vi "stateMachine_v2_Nov2015.vi"() -> ()   [LabVIEW 2014]
uses:
  daq_channel_read_parameter.ctl
  <vilib>/Platform/TimedLoop/XDataNode/timing_clust.ctl
  <vilib>/Platform/TimedLoop/XDataNode/nitl_modes.ctl
  <vilib>/Platform/TimedLoop/XDataNode/wakeup.ctl
  <vilib>/dex/Stream Element Allocation Mode.ctl
  states_def.ctl
  UDP_Para_def.ctl
  <vilib>/DAQmx/write.llb/DAQmx Write (Digital 1D Bool NChan 1Samp 1Line).vi
  <vilib>/platform/TimedLoop/XDataNode/XDataNode.xnode
  <vilib>/Platform/TimedLoop/XDataNode/XDNodeRunTimeDep.lvlib
  <resource>/objmgr/ni.dex.rc
panel:
  out "skipRewFlag":bool
  out "rightcounter":i32
  out "leftcounter":i32
  out "beh type":string
  out "vs type":string
  out "Tab Control":enum32{"State Machine"}(tab)
  in  "vsFilterPeriod_uS":i32=500 format="%#1.6f"
  in  "lickThreshold_V":fxp<+/-,16,5> format="%#.4g"
  in  "vsThreshold_V":fxp<+/-,16,5> format="%#.4g"
  in  "audioThreshold_V":fxp<+/-,16,5> format="%#.4g"
  in  "audioFilterPeriod_uS":i32=50000 format="%#1.6f"
  in  "audioOffState_V":fxp<+/-,16,5> format="%#.4g"
  out "rtFIFOsize":u32=50
  out "rtFIFOtimeout":u32
  out "rtFIFOdataPool":u32=50
  out "stateMachineCycle_uS":i64=500
  out "(Actual)":i64
  in  "delay_uS":u32
  out "IP_RT":string="192.168.137.2"
  in  "port_broadcast":u16=9091
  out "IP_host":string="192.168.137.1"
  out "port_host":u16=9090
  in  "Tab Control 2":enum32{"Data Transfer"}(tab)
  out "stream counter":u32
  out "Is Connected":bool
  out "Available Elements for Writing":i32
  out "stream writer buffer size":i32=500
  in  "rewardPeriod_uS":u32
  in  "waterOn_uS":u32
  in  "timeout_uS":u32=5000000
  in  "shockOn_uS":u32
  in  "Stop state":bool
  out "Initial data received":bool
  out "Tab Control 3":enum32{"Current status"}(tab)
  in  "toneReward":bool
  out "ABORT":bool
  out "trialStart":bool
  out "trialDone":bool
  out "Busy":bool
  out "stateLatched":bool
  out "curKey":u32=1
  out "curState":u32
  out "rtFIFOdataDim":i32
  in  "manualShock":bool
  in  "manualWaterRight":bool
  in  "manualWaterLeft":bool
  in  "lickReward":bool
  in  "allowPunish":bool
  in  "forceLRswitch":bool
  in  "allowCorrection":bool
  in  "allowAutoWater":bool
  out "error out":errorcluster
  in  "trialKey":i32[](array[numeric])
  in  "rwdrefPeriod_uS":u32
  out "FlagWaterLeft":bool
  in  "chanellParaCluster":T1={"audioOffState_V"=0.0, "audioFilterPeriod_uS"=50000, "audioThreshold_V"=0.0, "vsThreshold_V"=0.0, "vsFilterPeriod_uS"=0, "lickThreshold_V"=0.0} {"vsFilterPeriod_uS" format="%#1.6f"; "audioFilterPeriod_uS" format="%#1.6f"}
  out "leftWaterOnFlag":bool
  out "rightWaterOnFlag":bool
  out "contNoReward":i32
  out "rewardStatus":bool
types:
  T1 = typedef "daq_channel_read_parameter.ctl" = cluster{"audioOffState_V":fxp<+/-,16,5>, "audioFilterPeriod_uS":i32, "audioThreshold_V":fxp<+/-,16,5>, "vsThreshold_V":fxp<+/-,16,5>, "vsFilterPeriod_uS":i32, "lickThreshold_V":fxp<+/-,16,5>}
  T2 = typedef "XDNodeRunTimeDep.lvlib/timing_clust.ctl" = cluster{"Expected End [f-1]":u64, "Actual End [f-1]":u64, "Finished Late? [f-1]":bool, "Expected End [i-1]":u64, "Actual End [i-1]":u64, "Finished Late? [i-1]":bool, "Expected Start [i]":u64, "Actual Start [i]":u64, "Expected Start [f]":u64, "Actual Start [f]":u64, "Source Name":string, "Structure Name":string, "Period":i64, "Deadline":i64, "Offset":i64, "Start":i64, "Priority":i32, "Timeout":i32, "Mode":T3, "Wakeup Reason":T4, "Error":errorcluster, "Source Type":string, "Secondary Source Type":string, "Global End Time":u64, "Global Start Time":u64, "Frame Duration":u64, "Iteration Duration":u64, "Assigned CPU":i32, "I/O Scan Engine Mode":u32}
  T3 = typedef "XDNodeRunTimeDep.lvlib/nitl_modes.ctl" = enum32{"No Change", "Process missed periods, maintain original phase", "Discard missed periods, maintain original phase", "Process missed periods, ignore original phase", "Discard missed periods, ignore original phase"}
  T4 = typedef "XDNodeRunTimeDep.lvlib/wakeup.ctl" = enum32{"Normal", "Aborted", "Asynchronous wakeup", "Timing source error", "Timed loop error", "Timeout"}
  T5 = typedef "states_def.ctl" = enum16{"idle", "vs before", "vs", "vs after", "delay", "tone before", "tone", "tone after", "cycle end", "reward", "reward refractory", "punish", "punish refractory", "timeout", "exit", "manualwater"}
  T6 = typedef "Stream Element Allocation Mode.ctl" = u32
  T7 = typedef "UDP_Para_def.ctl" = enum16{"no", "start", "stop", "dly", "rwp", "rwf", "wdr", "shd", "tod", "lkr", "tlr", "alp", "msh", "mwl", "mwr", "alc", "lth", "vth", "ath", "aof", "afp", "vfp"}
  T8 = cluster{"leftLick":bool, "rightLick":bool, "visualStimuli2":bool, "tone":bool, "visualStimuli1":bool}
  T9 = cluster{"leftLick":dbl, "rightLick":dbl, "visualStimuli2":dbl, "tone":dbl, "visualStimuli1":dbl}
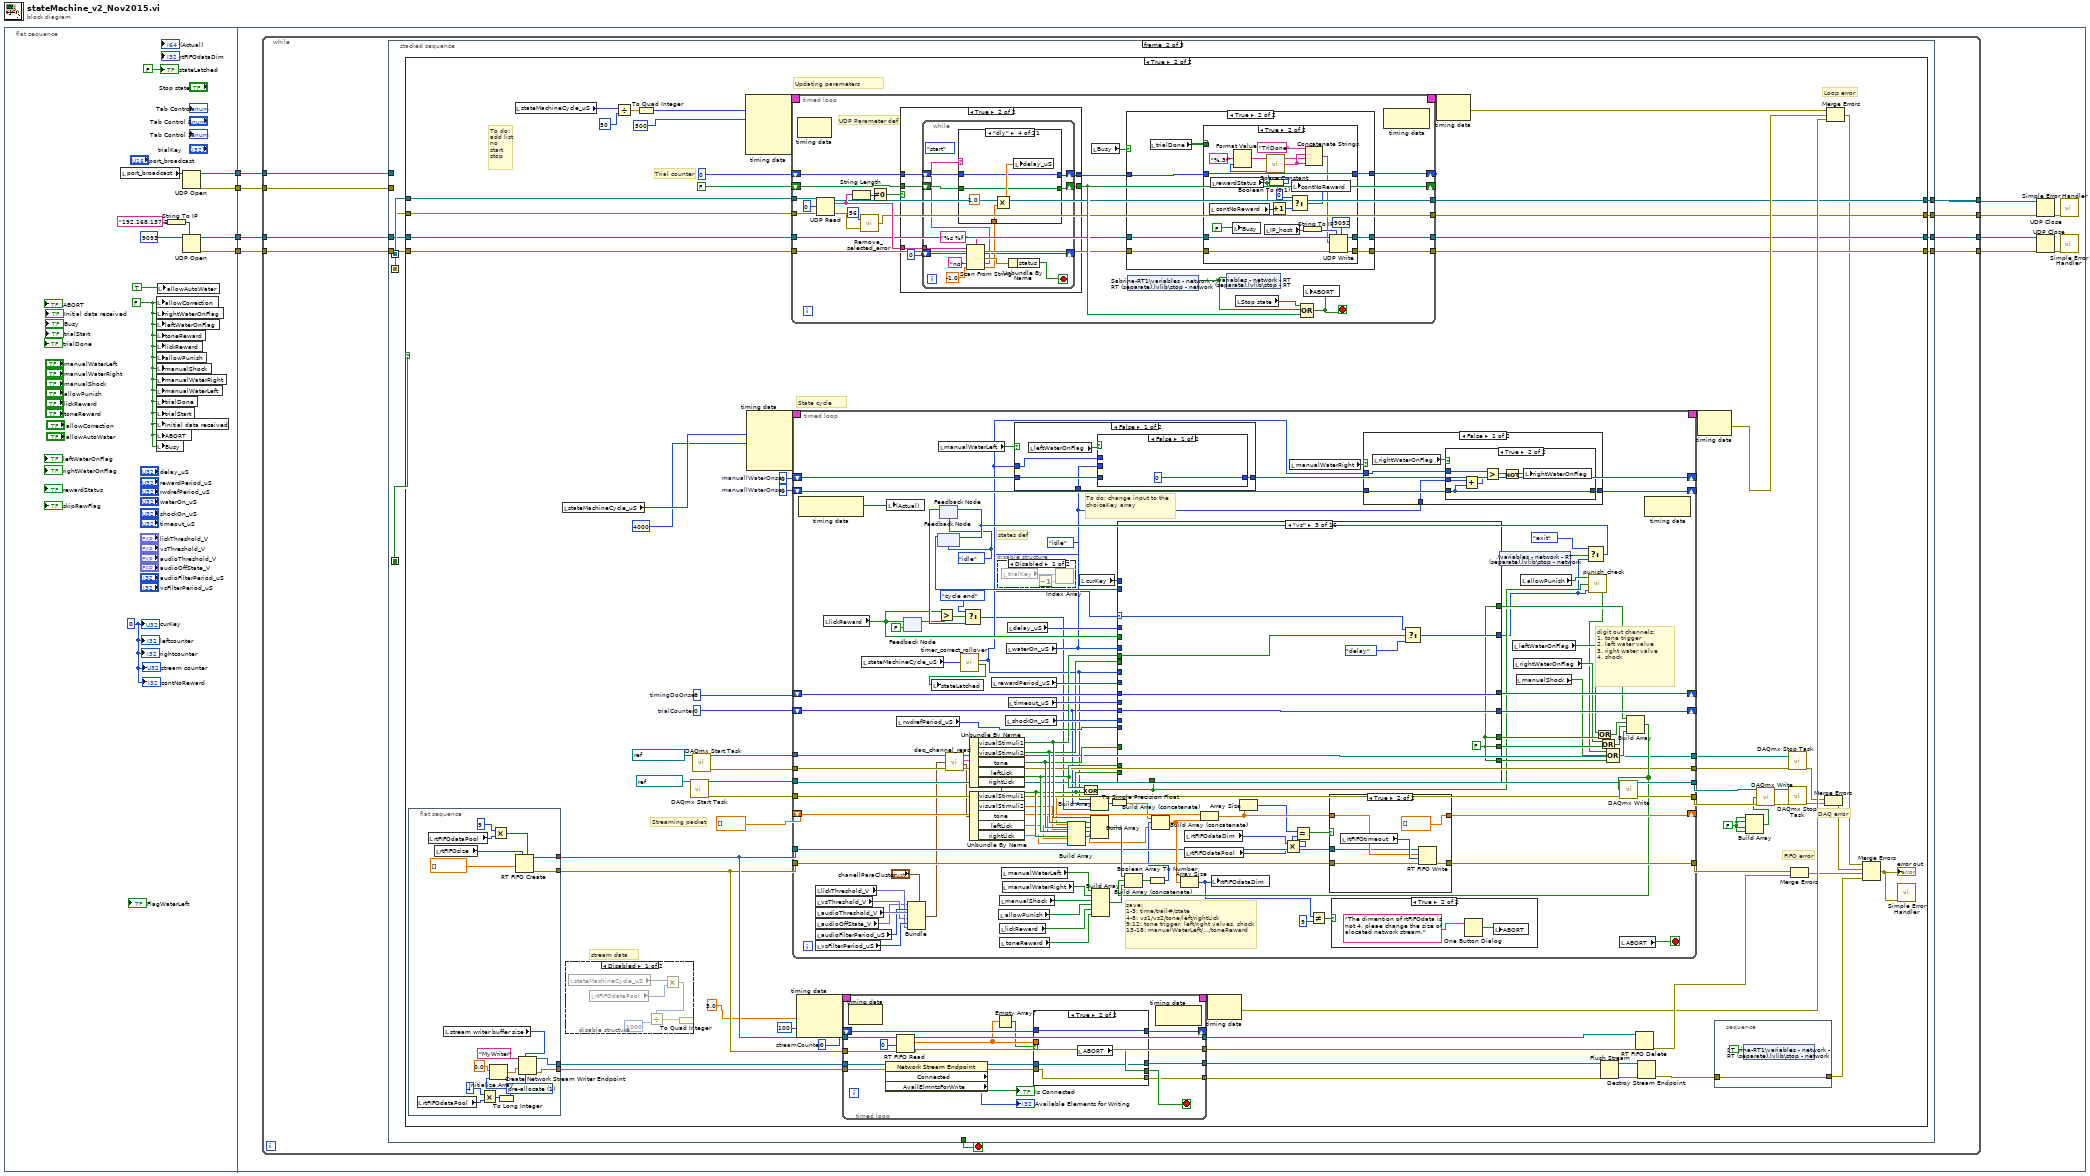
[diagram p0: block diagram]
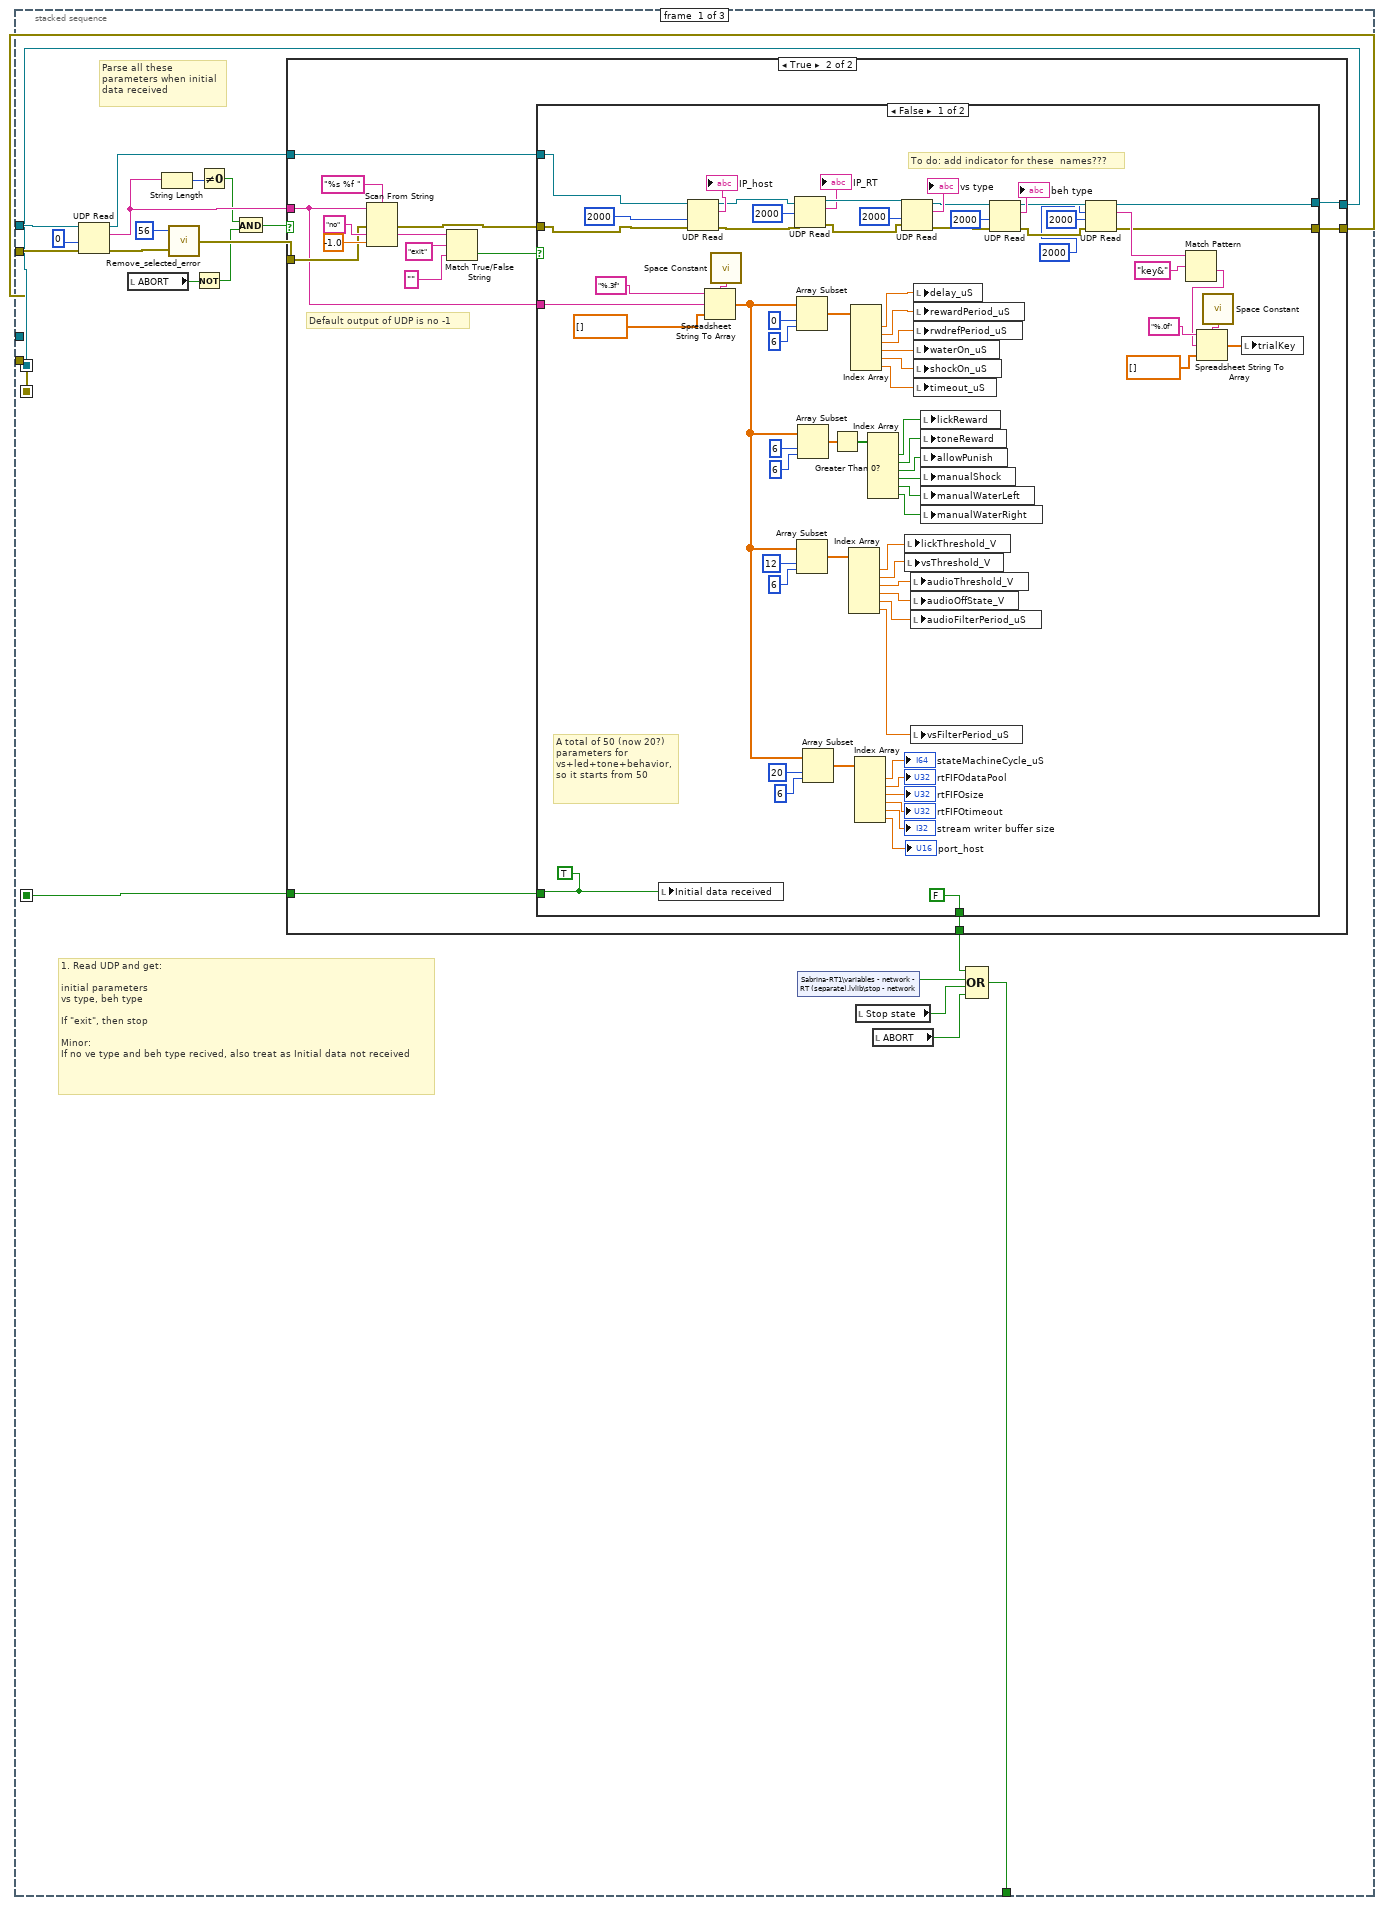
[diagram p2: hidden frame]
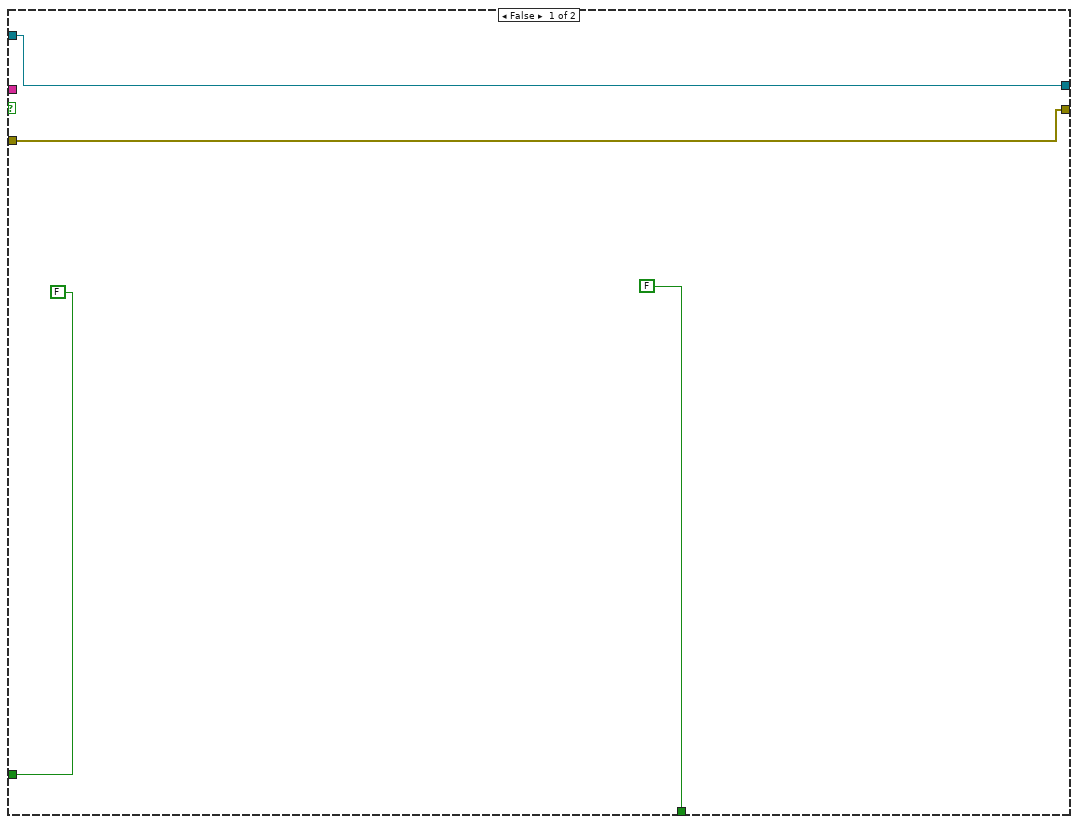
[diagram p3: hidden frame]
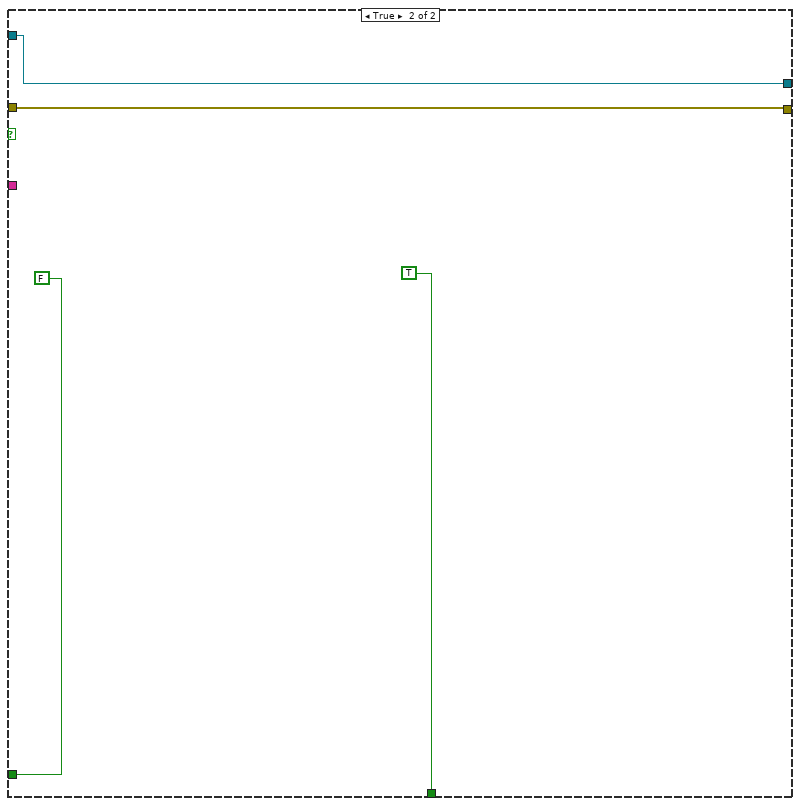
[diagram p4: hidden frame]
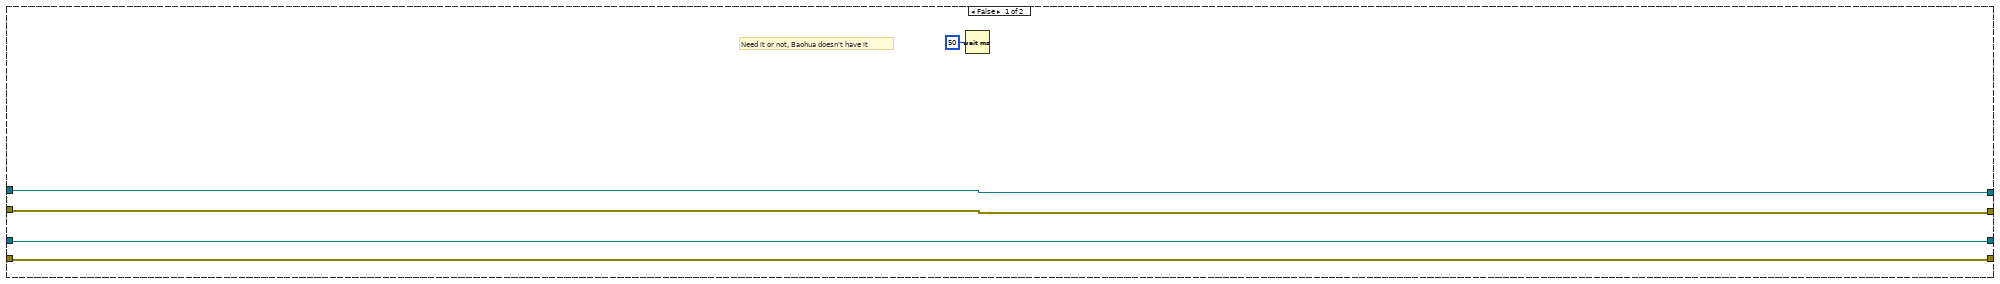
[diagram p5: hidden frame]
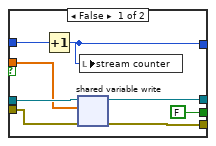
[diagram p7: hidden frame]
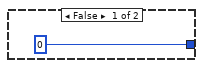
[diagram p9: hidden frame]
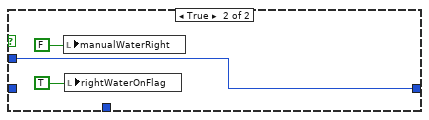
[diagram p10: hidden frame]
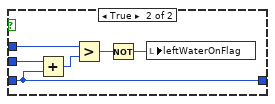
[diagram p11: hidden frame]
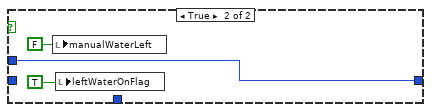
[diagram p12: hidden frame]
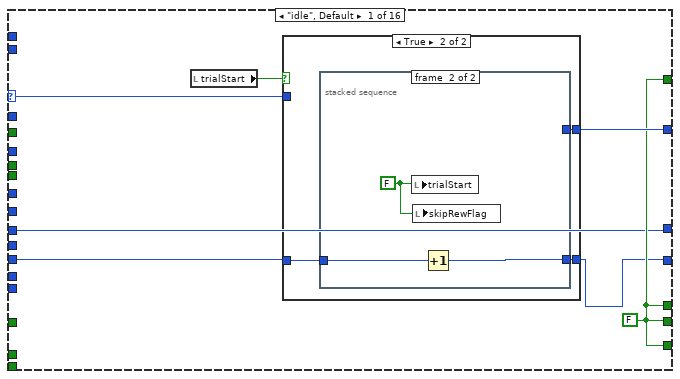
[diagram p15: hidden frame]
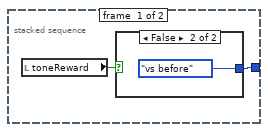
[diagram p17: hidden frame]
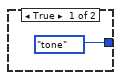
[diagram p18: hidden frame]
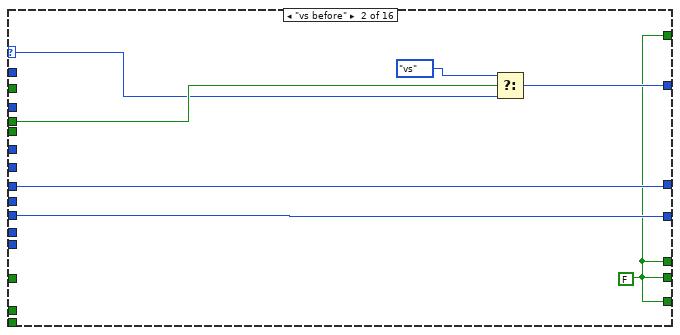
[diagram p19: hidden frame]
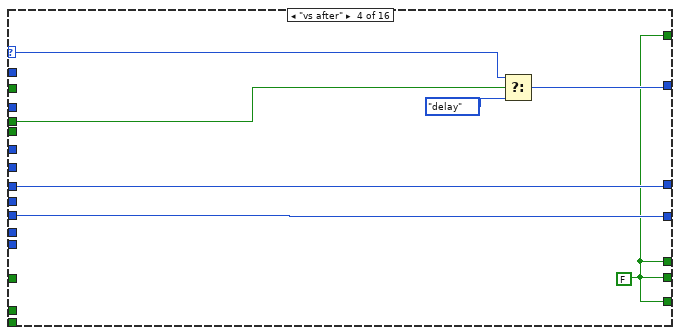
[diagram p20: hidden frame]
diagram:
  n1 = flat-sequence {
    tunnel: [w16] -> w4
    tunnel: [w15] -> w3
    tunnel: [w11] -> w2
    tunnel: [w10] -> w1
    tunnel: w4 -> [w26]
    tunnel: w3 -> [w25]
    tunnel: w2 -> [w21]
    tunnel: w1 -> [w20]
    frame #0 {
      w7 = FALSE
      w6 = 0
      n2 = local read "port_broadcast"() -> (w14:u16)
      n3 = local write "allowCorrection"(w7) -> ()
      n4 = local write "rightWaterOnFlag"(w7) -> ()
      n5 = local write "leftWaterOnFlag"(w7) -> ()
      n6 = local write "toneReward"(w7) -> ()
      n7 = local write "lickReward"(w7) -> ()
      n8 = local write "allowPunish"(w7) -> ()
      n9 = local write "manualShock"(w7) -> ()
      n10 = local write "manualWaterRight"(w7) -> ()
      n11 = local write "manualWaterLeft"(w7) -> ()
      n12 = local write "trialDone"(w7) -> ()
      n13 = local write "trialStart"(w7) -> ()
      n14 = local write "Initial data received"(w7) -> ()
      n15 = local write "ABORT"(w7) -> ()
      n16 = local write "Busy"(w7) -> ()
      n17 = local write "allowAutoWater"(TRUE) -> ()
      n18 = String To IP(1:"192.168.137.2") -> (0:w8:u32)
      n19 = UDP Open(7:w8, 11:u16 9093) -> (port=w11:refnum<k16>, 0:w10:errorcluster)  [unwired: 3 in, 1 out]
      n20 = UDP Open(11:w14) -> (port=w16:refnum<k16>, 0:w15:errorcluster)  [unwired: 4 in, 1 out]
      "stateLatched" <- FALSE
      "curKey" <- w6
      "leftcounter" <- w6
      "rightcounter" <- w6
      "stream counter" <- w6
      "contNoReward" <- w6
    }
    frame #1 {
      n21 = while {
        tunnel: w26 -> [w35]
        tunnel: w25 -> [w34]
        tunnel: [w32] -> w23
        tunnel: [w31] -> w22
        tunnel: w21 -> [w30]
        tunnel: w20 -> [w29]
        tunnel: [w28] -> w19
        tunnel: [w27] -> w18
        stop <- w33 stop-if-true
        n22 = stacked-sequence {
          seq-local: [w45 _ _] -> [_ w161 _]
          seq-local: [w37 _ _] -> [_ w158 _]
          seq-local: [w36 _ _] -> [_ w157 _]
          tunnel: w35 -> [w56 _ _]
          tunnel: w34 -> [w55 _ _]
          tunnel: [w46 _ _] -> w33
          tunnel: [_ w160 _] -> w32
          tunnel: [_ w159 _] -> w31
          tunnel: w30 -> [_ w156 _]
          tunnel: w29 -> [_ w153 _]
          tunnel: [_ w155 _] -> w28
          tunnel: [_ w154 _] -> w27
          frame #0 {
            # "Parse all these \nparameters when initial\ndata received"
            # "1. Read UDP and get:\n\ninitial parameters\nvs type, beh type\n\nIf \"exit\", then stop\n\nMinor:\nIf no ve type and beh type recived, also treat as Initial data not received"
            n23 = UDP Read(connection ID=w56, timeout ms (25000)=0, 8:w55) -> (data out=w53:string, error out=w43:errorcluster, 3:w54:refnum<k16>)  [unwired: 1 in, 2 out]
            n24 = local read "ABORT"() -> (w41:bool)
            n25 = String Length(string=w53) -> (length=w52:i32)
            n26 = call "Remove_selected_error.vi"("error in (no error)"=w43, "errorCode"=56 ("timeout ms (25000)")) -> ("error out"=w44:errorcluster)
            n27 = Not(x=w41) -> (.not. x?=w38:bool)
            n28 = Not Equal To 0?(x=w52) -> (x != 0?=w39:bool)
            n29 = And(x=w39, y=w38) -> (x .and. y?=w40:bool)
            n30 = case shown="True" w40 {
              tunnel: w53 -> [_ w65]
              tunnel: w54 -> [w58 w66]
              tunnel: w44 -> [w57 w73]
              tunnel: [FALSE w64] -> w50
              tunnel: [FALSE w63] -> w45
              tunnel: [w58 w62] -> w37
              tunnel: [w57 w61] -> w36
              frame False {
              }
              frame True {
                # "Default output of UDP is no -1"
                n31 = Scan From String(format string="%s %f ", input string=w65, error in=w73, default 1="no" ("default value 1"), default 2=sgl -1.0 ("default value 1")) -> (error out=w67:errorcluster, output 1=w72:string)  [unwired: 2 in, 2 out]
                n32 = Match True/False String(2:"" ("false string"), 3:"exit" ("true string"), 4:w72) -> (0:w68:bool)  [unwired: 1 out]
                n33 = case shown="False" w68 {
                  tunnel: w67 -> [w110 w150]
                  tunnel: w66 -> [w111 w149]
                  tunnel: w65 -> [w142 _]
                  tunnel: [FALSE TRUE] -> w64
                  tunnel: [w140 FALSE] -> w63
                  tunnel: [w77 w149] -> w62
                  tunnel: [w76 w150] -> w61
                  frame False {
                    w140 = TRUE
                    # "A total of 50 (now 20?) parameters for vs+led+tone+behavior, so it starts from 50"
                    # "To do: add indicator for these  names???"
                    n34 = local write "Initial data received"(w140) -> ()
                    n35 = UDP Read(connection ID=w111, timeout ms (25000)=2000, 8:w110) -> (data out=→"IP_host":string, error out=w109:errorcluster, 3:w107:refnum<k16>)  [unwired: 1 in, 2 out]
                    n36 = call <vilib>:"Space Constant.vi"() -> ("String"=w147:string)
                    n37 = Spreadsheet String To Array(delimiter (Tab)=w147, format string="%.3f", spreadsheet string=w142, array type (2D Dbl)=sgl[] []) -> (array=w118:sgl[])
                    n38 = UDP Read(connection ID=w107, timeout ms (25000)=2000, 8:w109) -> (data out=→"IP_RT":string, error out=w108:errorcluster, 3:w106:refnum<k16>)  [unwired: 1 in, 2 out]
                    n39 = Array Subset(array=w118, index=0 ("timeout ms (25000)"), length=6 ("timeout ms (25000)")) -> (w136:sgl[])
                    n40 = Array Subset(array=w118, index=12 ("timeout ms (25000)"), length=6 ("timeout ms (25000)")) -> (w132:sgl[])
                    n41 = Array Subset(array=w118, index=6 ("timeout ms (25000)"), length=6 ("timeout ms (25000)")) -> (w129:sgl[])
                    n42 = Array Subset(array=w118, index=20 ("timeout ms (25000)"), length=6 ("timeout ms (25000)")) -> (w119:sgl[])
                    n43 = Greater Than 0?(x=w129) -> (x > 0?=w128:bool[])
                    n44 = Index Array(array=w132) -> (element #1=w94:sgl, element #2=w93:sgl, element #3=w92:sgl, element #4=w91:sgl, element #5=w90:sgl, element #6=w89:sgl)  [unwired: 6 in]
                    n45 = Index Array(array=w136) -> (element #1=w100:sgl, element #2=w99:sgl, element #3=w98:sgl, element #4=w97:sgl, element #5=w96:sgl, element #6=w95:sgl)  [unwired: 6 in]
                    n46 = Index Array(array=w119) -> (element #1=→"stateMachineCycle_uS":sgl, element #2=→"rtFIFOdataPool":sgl, element #3=→"rtFIFOsize":sgl, element #4=→"rtFIFOtimeout":sgl, element #5=→"stream writer buffer size":sgl, element #6=→"port_host":sgl)  [unwired: 6 in]
                    n47 = Index Array(array=w128) -> (element #1=w127:bool, element #2=w126:bool, element #3=w125:bool, element #4=w124:bool, element #5=w123:bool, element #6=w122:bool)  [unwired: 6 in]
                    n48 = UDP Read(connection ID=w106, timeout ms (25000)=2000, 8:w108) -> (data out=→"vs type":string, error out=w139:errorcluster, 3:w138:refnum<k16>)  [unwired: 1 in, 2 out]
                    n49 = local write "lickThreshold_V"(w94) -> ()
                    n50 = local write "vsThreshold_V"(w93) -> ()
                    n51 = local write "audioThreshold_V"(w92) -> ()
                    n52 = local write "audioOffState_V"(w91) -> ()
                    n53 = local write "audioFilterPeriod_uS"(w90) -> ()
                    n54 = local write "vsFilterPeriod_uS"(w89) -> ()
                    n55 = local write "delay_uS"(w100) -> ()
                    n56 = local write "rewardPeriod_uS"(w99) -> ()
                    n57 = local write "rwdrefPeriod_uS"(w98) -> ()
                    n58 = local write "waterOn_uS"(w97) -> ()
                    n59 = local write "shockOn_uS"(w96) -> ()
                    n60 = local write "timeout_uS"(w95) -> ()
                    n61 = local write "lickReward"(w127) -> ()
                    n62 = local write "toneReward"(w126) -> ()
                    n63 = local write "allowPunish"(w125) -> ()
                    n64 = local write "manualShock"(w124) -> ()
                    n65 = local write "manualWaterLeft"(w123) -> ()
                    n66 = local write "manualWaterRight"(w122) -> ()
                    n67 = UDP Read(connection ID=w138, timeout ms (25000)=2000, 8:w139) -> (data out=→"beh type":string, error out=w86:errorcluster, 3:w87:refnum<k16>)  [unwired: 1 in, 2 out]
                    n68 = UDP Read(connection ID=w87, max size (548)=2000 ("timeout ms (25000)"), timeout ms (25000)=2000, 8:w86) -> (data out=w81:string, error out=w76:errorcluster, 3:w77:refnum<k16>)  [unwired: 2 out]
                    n69 = Match Pattern(string=w81, regular expression="key&") -> (after substring=w79:string)  [unwired: 1 in, 3 out]
                    n70 = call <vilib>:"Space Constant.vi"() -> ("String"=w84:string)
                    n71 = Spreadsheet String To Array(delimiter (Tab)=w84, format string="%.0f", spreadsheet string=w79, array type (2D Dbl)=dbl[] []) -> (array=w82:dbl[])
                    n72 = local write "trialKey"(w82) -> ()
                  }
                  frame True {
                  }
                }
              }
            }
            n73 = shared-variable "Sabrina-RT1\\variables - network - RT (separate).lvlib\\stop - network"() -> (w49:bool)  [unwired: 1 in, 1 out]
            n74 = local read "Stop state"() -> (w48:bool)
            n75 = local read "ABORT"() -> (w47:bool)
            n76 = Compound Arithmetic op=OR(w50, w49, w48, w47) -> (w46:bool)
          }
          frame #1 {
            n77 = case shown="True" w161 {
              tunnel: w158 -> [w165 w211]
              tunnel: w157 -> [w164 w210]
              tunnel: [w165 w183] -> w160
              tunnel: [w164 w184] -> w159
              tunnel: w156 -> [w163 w188]
              tunnel: w153 -> [w162 w187]
              tunnel: [w162 w186] -> w155
              tunnel: [w163 w185] -> w154
              frame False {
                # "Need it or not, Baohua doesn't have it"
                n78 = Wait (ms)(milliseconds to wait=u32 50) -> ()  [unwired: 1 out]
              }
              frame True {
                w167 = 0  # manuallWaterOnset
                w168 = 0  # manuallWaterOnset
                w194 = FALSE
                w223 = 0  # streamCounter
                w226 = 0  # timingDoOnset
                w225 = 0  # trialCounter
                # "Streaming packet"
                # "Trial counter"
                # "Loop error"
                # "DAQ error"
                # "FIFO error"
                # "Updating parameters"
                # "State cycle"
                # "To do:\nadd list\nno\nstart\nstop"
                # "stream data"
                n79 = flat-sequence {
                  tunnel: [w253] -> w228
                  tunnel: [w252] -> w227
                  tunnel: [w251] -> w214
                  tunnel: [w250] -> w213
                  frame #0 {
                    w257 = T6 1 items=["allocate as needed", "pre-allocate"] ("element allocation mode")
                    n80 = local read "rtFIFOdataPool"() -> (w248:u32)
                    n81 = local read "rtFIFOdataPool"() -> (w245:u32)
                    n82 = local read "rtFIFOsize"() -> (w259:u32)
                    n83 = local read "stream writer buffer size"() -> (w249:i32)
                    n84 = Multiply(x=u32 4, y=w248) -> (x*y=w243:u32)
                    n85 = Multiply(x=9, y=w245) -> (x*y=w244:u32)
                    n86 = To Long Integer(number=w243) -> (32bit integer=w242:i32)
                    n87 = Initialize Array(sgl 0.0, w242) -> (w256:sgl[])
                    n88 = RT FIFO Create(1:sgl[] [], 4:w259, 6:w244) -> (8:w251:refnum<k33>, 11:w250:errorcluster)  [unwired: 5 in, 1 out]
                    n89 = Create Network Stream Writer Endpoint(6:w257, 7:w249, 9:w256, 11:"MyWriter" ("writer name")) -> (0:w253:errorcluster, 3:w252:refnum<k21>)  [unwired: 3 in]
                  }
                }
                n90 = local read "stateMachineCycle_uS"() -> (w212:i64)
                n91 = local read "stateMachineCycle_uS"() -> (w222:i64)
                n92 = disable-structure shown="Disabled" {
                  frame Disabled {
                    n93 = local read "stateMachineCycle_uS"() -> (w237:i64)
                    n94 = local read "rtFIFOdataPool"() -> (w236:u32)
                    n95 = Multiply(x=w237, y=w236) -> (x*y=w238:i64)
                    n96 = Divide(x=w238, y=i64 1000) -> (x/y=w235:dbl)
                    n97 = To Quad Integer(1:w235) -> ()  [unwired: 1 out]
                  }
                  frame Enabled {
                  }
                }
                n98 = Divide(x=w212, y=i64 50) -> (x/y=w218:dbl)
                n99 = To Quad Integer(1:w218) -> (0:w217:i64)
                n100 = call <vilib>:"DAQmx Start Task.vi"("task/channels in"=refnum<k21> "digitWrite" ("digitWrite")) -> ("task out"=w180:refnum<k21>, "error out"=w179:errorcluster)  [unwired: 13 in]
                n101 = call <vilib>:"DAQmx Start Task.vi"("task/channels in"=refnum<k21> "analogRead" ("DAQmx Task Name")) -> ("task out"=w170:refnum<k21>, "error out"=w169:errorcluster)  [unwired: 13 in]
                n102 = node-c288(w217, 500 ("Priority")) -> (w234:T2)  [unwired: 3 in]
                n103 = node-c288(w222, 4000 ("Priority")) -> (w232:T2)  [unwired: 3 in]
                n104 = timed-loop {
                  timing: w234 -> [_]
                  timing-out: [_] -> w233
                  shift-right: [w743] -> _
                  shift-left: 0 ("timeout ms (25000)") -> [w745]
                  shift-right: [w739] -> _
                  shift-left: FALSE -> [w742]
                  tunnel: [w736] -> w185
                  tunnel: [w735] -> w186
                  tunnel: w211 -> [w734]
                  tunnel: w210 -> [w733]
                  tunnel: w188 -> [w727]
                  tunnel: w187 -> [w730]
                  tunnel: [w729] -> w184
                  tunnel: [w728] -> w183
                  stop <- w741 stop-if-true
                  # "UDP Parameter def"
                  n105 = node-c288() -> ()  [unwired: 1 in, 1 out]
                  n106 = UDP Read(connection ID=w734, timeout ms (25000)=0, 8:w733) -> (data out=w746:string, error out=w732:errorcluster, 3:w728:refnum<k16>)  [unwired: 1 in, 2 out]
                  n107 = String Length(string=w746) -> (length=w748:i32)
                  n108 = call "Remove_selected_error.vi"("error in (no error)"=w732, "errorCode"=56 ("timeout ms (25000)")) -> ("error out"=w729:errorcluster)
                  n109 = Not Equal To 0?(x=w748) -> (x != 0?=w747:bool)
                  n110 = case shown="True" w747 {
                    tunnel: w746 -> [_ w790]
                    tunnel: w745 -> [w784 w789]
                    tunnel: [w784 w788] -> w744
                    tunnel: w742 -> [w783 w787]
                    tunnel: [w783 w786] -> w739
                    frame False {
                    }
                    frame True {
                      n111 = while {
                        tunnel: w790 -> [w804]
                        shift-right: [w791] -> _
                        shift-left: 0 ("timeout ms (25000)") -> [w792]
                        shift-right: [w797] -> w788
                        shift-left: w789 -> [w798]
                        shift-right: [w795] -> w786
                        shift-left: w787 -> [w796]
                        stop <- w799 stop-if-true
                        (unwired) UDP_Para_def."start"
                        n112 = Scan From String(format string="%s %f ", input string=w804, initial scan location=w792, default 1="no" ("default value 1"), default 2=-1.0 ("default value 2")) -> (offset past scan=w791:u32, error out=w800:errorcluster, output 1=w794:string, output 2=w793:dbl)  [unwired: 1 in, 1 out]
                        n113 = case shown="\"dly\"" w794 {
                          tunnel: [w806 w808 w817 w819 w824 w829 w834 w839 w844 w849 w853 w857 w861 w865 w869 w873 w877 w881 w885 w889 w894] -> w797
                          tunnel: w798 -> [w806 w809 w817 w819 w824 w829 w834 w839 w844 w849 w853 w857 w861 w865 w869 w873 w877 w881 w885 w889 w894]
                          tunnel: [w805 w813 w814 w818 w823 w828 w833 w838 w843 w848 w852 w856 w860 w864 w868 w872 w876 w880 w884 w888 w893] -> w795
                          tunnel: w796 -> [w805 w813 w815 w818 w823 w828 w833 w838 w843 w848 w852 w856 w860 w864 w868 w872 w876 w880 w884 w888 w893]
                          tunnel: w793 -> [_ w810 _ w821 w826 w831 w836 w841 w846 w851 w855 w859 w863 w867 w871 w875 w879 w883 w887 w891 w896]
                          frame "no", Default {
                          }
                          frame "start" {
                            w812 = TRUE
                            n114 = Increment(x=w809) -> (x+1=w808:i32)
                            n115 = local write "rewardStatus"(FALSE) -> ()
                            n116 = local write "trialDone"(FALSE) -> ()
                            n117 = local write "Busy"(w812) -> ()
                            n118 = local write "trialStart"(w812) -> ()
                            n119 = local write "curKey"(w810) -> ()
                          }
                          frame "stop" {
                            n120 = Or(x=w815, y=TRUE) -> (x .or. y?=w814:bool)
                          }
                          frame "dly" {
                            n121 = Multiply(x=1.0, y=w821) -> (x*y=w820:dbl)
                            n122 = local write "delay_uS"(w820) -> ()
                          }
                          frame "rwp" {
                            n123 = Multiply(x=1.0, y=w826) -> (x*y=w825:dbl)
                            n124 = local write "rewardPeriod_uS"(w825) -> ()
                          }
                          frame "rwf" {
                            n125 = Multiply(x=1.0, y=w831) -> (x*y=w830:dbl)
                            n126 = local write "rwdrefPeriod_uS"(w830) -> ()
                          }
                          frame "wdr" {
                            n127 = Multiply(x=1.0, y=w836) -> (x*y=w835:dbl)
                            n128 = local write "waterOn_uS"(w835) -> ()
                          }
                          frame "shd" {
                            n129 = Multiply(x=1.0, y=w841) -> (x*y=w840:dbl)
                            n130 = local write "shockOn_uS"(w840) -> ()
                          }
                          frame "tod" {
                            n131 = Multiply(x=1.0, y=w846) -> (x*y=w845:dbl)
                            n132 = local write "timeout_uS"(w845) -> ()
                          }
                          frame "lkr" {
                            n133 = Greater Than 0?(x=w851) -> (x > 0?=w850:bool)
                            n134 = local write "lickReward"(w850) -> ()
                          }
                          frame "tlr" {
                            n135 = Greater Than 0?(x=w855) -> (x > 0?=w854:bool)
                            n136 = local write "toneReward"(w854) -> ()
                          }
                          frame "alp" {
                            n137 = Greater Than 0?(x=w859) -> (x > 0?=w858:bool)
                            n138 = local write "allowPunish"(w858) -> ()
                          }
                          frame "msh" {
                            n139 = Greater Than 0?(x=w863) -> (x > 0?=w862:bool)
                            n140 = local write "manualShock"(w862) -> ()
                          }
                          frame "mwl" {
                            n141 = Greater Than 0?(x=w867) -> (x > 0?=w866:bool)
                            n142 = local write "manualWaterLeft"(w866) -> ()
                          }
                          frame "mwr" {
                            n143 = Greater Than 0?(x=w871) -> (x > 0?=w870:bool)
                            n144 = local write "manualWaterRight"(w870) -> ()
                          }
                          frame "lth" {
                            n145 = To Fixed-Point(number=w875) -> (fixed-point=w874:fxp<+/-,32,16>)  [unwired: 1 in]
                            n146 = local write "lickThreshold_V"(w874) -> ()
                          }
                          frame "vth" {
                            n147 = To Fixed-Point(number=w879) -> (fixed-point=w878:fxp<+/-,32,16>)  [unwired: 1 in]
                            n148 = local write "vsThreshold_V"(w878) -> ()
                          }
                          frame "ath" {
                            n149 = To Fixed-Point(number=w883) -> (fixed-point=w882:fxp<+/-,32,16>)  [unwired: 1 in]
                            n150 = local write "audioThreshold_V"(w882) -> ()
                          }
                          frame "aof" {
                            n151 = To Fixed-Point(number=w887) -> (fixed-point=w886:fxp<+/-,32,16>)  [unwired: 1 in]
                            n152 = local write "audioOffState_V"(w886) -> ()
                          }
                          frame "afp" {
                            n153 = Multiply(x=1.0, y=w891) -> (x*y=w890:dbl)
                            n154 = local write "audioFilterPeriod_uS"(w890) -> ()
                          }
                          frame "vfp" {
                            n155 = Multiply(x=1.0, y=w896) -> (x*y=w895:dbl)
                            n156 = local write "vsFilterPeriod_uS"(w895) -> ()
                          }
                        }
                        n157 = Unbundle By Name(w800) -> ("status"=w799:bool)
                      }
                    }
                  }
                  n158 = local read "Busy"() -> (w740:bool)
                  n159 = case shown="True" w740 {
                    tunnel: w744 -> [w752 w759]
                    tunnel: [w752 w758] -> w743
                    tunnel: w727 -> [w751 w757]
                    tunnel: [w751 w756] -> w736
                    tunnel: [w750 w755] -> w735
                    tunnel: w730 -> [w750 w754]
                    frame False {
                    }
                    frame True {
                      n160 = local read "trialDone"() -> (w753:bool)
                      n161 = case shown="True" w753 {
                        tunnel: w759 -> [w762 w777]
                        tunnel: [w762 w777] -> w758
                        tunnel: w757 -> [w761 w776]
                        tunnel: [w761 w775] -> w756
                        tunnel: [w760 w774] -> w755
                        tunnel: w753 -> [_ _]
                        tunnel: w754 -> [w760 w771]
                        frame False {
                        }
                        frame True {
                          n162 = local read "contNoReward"() -> (w765:i32)
                          n163 = local read "rewardStatus"() -> (w767:bool)
                          n164 = local write "Busy"(FALSE) -> ()
                          n165 = local read "IP_host"() -> (w772:string)
                          n166 = call <vilib>:"Space Constant.vi"() -> ("String"=w781:string)
                          n167 = Boolean To (0,1)(Boolean=w767) -> (0, 1=w768:i16)
                          n168 = Format Value(format string="%.3f", value (0)=w768) -> (output string=w779:string)  [unwired: 1 in]
                          n169 = Increment(x=w765) -> (x+1=w764:i32)
                          n170 = Select(t=0 ("timeout ms (25000)"), s=w767, f=w764) -> (s? t:f=w763:i32)
                          n171 = local write "contNoReward"(w763) -> ()
                          n172 = String To IP(1:w772) -> (0:w778:u32)
                          n173 = Concatenate Strings("TrlDone" ("data in"), w781, w779, w781) -> (w770:string)
                          n174 = UDP Write(address=w778, port or service name=u16 9092, connection ID=w776, data in=w770, 8:w771) -> (error out=w774:errorcluster, 3:w775:refnum<k16>)  [unwired: 1 in]
                        }
                      }
                    }
                  }
                  n175 = shared-variable "Sabrina-RT1\\variables - network - RT (separate).lvlib\\stop - network"() -> (w738:bool)  [unwired: 1 in, 1 out]
                  n176 = shared-variable ".\\variables - network - RT (separate).lvlib\\stop - RT"(w738) -> ()  [unwired: 1 in, 1 out]
                  n177 = local read "Stop state"() -> (w737:bool)
                  n178 = Compound Arithmetic op=OR(w737, w738, w739) -> (w741:bool)
                  n179 = local write "ABORT"(w741) -> ()
                  n180 = node-c288() -> ()  [unwired: 1 in, 1 out]
                }
                n181 = timed-loop {
                  timing: w232 -> [_]
                  timing-out: [_] -> w231
                  shift-right: [w386] -> _
                  shift-left: w225 -> [w324]
                  tunnel: [w397] -> w201
                  tunnel: [w396] -> w200
                  shift-right: [w394] -> _
                  shift-left: w226 -> [w395]
                  tunnel: w170 -> [w388]
                  tunnel: w169 -> [w354]
                  tunnel: [w326] -> w175
                  shift-right: [w379] -> _
                  shift-left: sgl[] [] ("array type (2D Dbl)") -> [w380]
                  tunnel: [w376] -> w191
                  tunnel: w214 -> [w353]
                  tunnel: w213 -> [w352]
                  tunnel: w180 -> [w342]
                  tunnel: w179 -> [w341]
                  tunnel: [w336] -> w176
                  shift-right: [w314] -> _
                  shift-left: w168 -> [w315]
                  shift-right: [w310] -> _
                  shift-left: w167 -> [w311]
                  stop <- w337 stop-if-true
                  w346 = states_def."idle"
                  # "states def"
                  # "save: \n1-3: time/trail#/state\n4-8: vs1/vs2/tone/left/rightLick\n9:12: tone trigger, left/right valves, shock\n13-18: manualWaterLeft/.../toneReward"
                  # "digit out channels:\n1. tone trigger\n2. left water valve\n3. right water valve\n4. shock"
                  # "To do: change input to the choiceKey array"
                  n182 = node-c288() -> (w349:i64)  [unwired: 1 in]
                  n183 = local read "lickThreshold_V"() -> (w330:fxp<+/-,16,5>)
                  n184 = local read "vsThreshold_V"() -> (w329:fxp<+/-,16,5>)
                  n185 = local read "audioThreshold_V"() -> (w335:fxp<+/-,16,5>)
                  n186 = local read "audioOffState_V"() -> (w328:fxp<+/-,16,5>)
                  n187 = local read "audioFilterPeriod_uS"() -> (w331:i32)
                  n188 = local read "vsFilterPeriod_uS"() -> (w332:i32)
                  n189 = local read "lickReward"() -> (w355:bool)
                  n190 = local read "stateMachineCycle_uS"() -> (w350:i64)
                  n191 = local write "(Actual)"(w349) -> ()
                  n192 = local read "rwdrefPeriod_uS"() -> (w343:u32)
                  n193 = feedback #1(FALSE ("lick-reward")) -> (w400:bool)
                  n194 = feedback-in #1(w355) -> ()
                  n195 = Bundle(cluster="chanellParaCluster", "audioOffState_V"=w328, "audioFilterPeriod_uS"=w331, "audioThreshold_V"=w335, "vsThreshold_V"=w329, "vsFilterPeriod_uS"=w332, "lickThreshold_V"=w330) -> (w334:T1)
                  n196 = feedback #2(w346) -> (w398:u32)
                  n197 = Greater?(x=w355, y=w400) -> (0:w401:bool)
                  n198 = local read "manualWaterLeft"() -> (w316:bool)
                  n199 = feedback #3(w346) -> (w402:u32)
                  n200 = call "daq_channel_read.vi"("DAQmxTaskIn"=w388, "chanellParaCluster"=w334, "error in (no error)"=w354) -> ("DAQmxTaskOut"=w336:refnum<k21>, "channelOutCluster"=w327:T8, "channelOutCluster_rawData"=w325:T9, "error out"=w326:errorcluster)
                  n201 = call "timer_correct_rollover.vi"("Loop Rate(uSec)"=w350) -> ("Late? (Latched)"=w389:bool, "Tick Count(uSec)"=w309:u64)  [unwired: 8 in, 1 out]
                  n202 = local write "stateLatched"(w389) -> ()
                  n203 = Select(t=states_def."cycle end", s=w401, f=w402) -> (s? t:f=w299:u32)
                  n204 = Unbundle By Name(w327) -> ("visualStimuli1"=w385:bool, "visualStimuli2"=w384:bool, "tone"=w383:bool, "leftLick"=w382:bool, "rightLick"=w381:bool)
                  n205 = Unbundle By Name(w325) -> ("visualStimuli1"=w318:dbl, "visualStimuli2"=w323:dbl, "tone"=w322:dbl, "leftLick"=w321:dbl, "rightLick"=w320:dbl)
                  n206 = local read "rewardPeriod_uS"() -> (w392:u32)
                  n207 = disable-structure shown="Disabled" {
                    frame Disabled {
                      n208 = local read "trialKey"() -> (w405:i32[])
                      n209 = Decrement() -> (x-1=w404:dbl)  [unwired: 1 in]
                      n210 = Index Array(array=w405, index=w404) -> ()  [unwired: 1 out]
                    }
                    frame Enabled {
                    }
                  }
                  n211 = local read "allowPunish"() -> (w364:bool)
                  n212 = local read "manualShock"() -> (w363:bool)
                  n213 = local read "lickReward"() -> (w365:bool)
                  n214 = local read "toneReward"() -> (w344:bool)
                  n215 = local read "manualWaterLeft"() -> (w362:bool)
                  n216 = local read "manualWaterRight"() -> (w361:bool)
                  n217 = local read "shockOn_uS"() -> (w387:u32)
                  n218 = local read "waterOn_uS"() -> (w308:u32)
                  n219 = local read "delay_uS"() -> (w345:u32)
                  n220 = local read "timeout_uS"() -> (w391:u32)
                  n221 = case shown="False" w316 {
                    tunnel: w315 -> [w424 _]
                    tunnel: [w423 w435] -> w314
                    tunnel: w309 -> [w422 w435]
                    tunnel: w308 -> [w421 _]
                    frame False {
                      n222 = local read "leftWaterOnFlag"() -> (w425:bool)
                      n223 = case shown="False" w425 {
                        tunnel: w424 -> [_ w430]
                        tunnel: [0 w430] -> w423
                        tunnel: w422 -> [_ w432]
                        tunnel: w421 -> [_ w431]
                        frame False {
                        }
                        frame True {
                          n224 = Add(x=w431, y=w430) -> (x+y=w429:u64)
                          n225 = Greater?(x=w432, y=w429) -> (0:w428:bool)
                          n226 = Not(x=w428) -> (.not. x?=w427:bool)
                          n227 = local write "leftWaterOnFlag"(w427) -> ()
                        }
                      }
                    }
                    frame True {
                      n228 = local write "manualWaterLeft"(FALSE) -> ()
                      n229 = local write "leftWaterOnFlag"(TRUE) -> ()
                    }
                  }
                  n230 = Build Array(w318, w323, w322, w321, w320) -> (w317:dbl[])
                  n231 = local read "curKey"() -> (w306:u32)
                  n232 = Exclusive Or(1:w381, 2:w382) -> (0:w302:bool)
                  n233 = Build Array(w309, w324, w299) -> (w359:u64[])
                  n234 = Build Array(w385, w384, w383, w382, w381) -> (w369:bool[])
                  n235 = Build Array(w362, w361, w363, w364, w365, w344) -> (w368:bool[])
                  n236 = To Single Precision Float(number=w359) -> (single precision float=w360:sgl[])
                  n237 = case shown="\"vs\"" states_def."idle" {
                    selector: states_def."idle" -> [w449 w469 w477 w485 w498 w514 w527 w536 w615 w634 w669 w677 w691 w702 w708 _]
                    tunnel: w385 -> [_ w471 w478 w484 _ _ _ _ _ _ _ _ _ _ _ _]
                    tunnel: w398 -> [_ _ _ _ w499 _ _ _ _ w652 _ w683 _ w703 _ _]
                    tunnel: w309 -> [_ _ _ _ w501 w509 w523 w551 w618 w650 w666 w678 _ w700 _ _]
                    tunnel: [w452 w470 w476 w483 w504 w508 w528 w550 w622 w648 w670 w681 w691 w701 w708 states_def."tone after"] -> w301
                    tunnel: w384 -> [_ _ _ _ _ _ _ _ _ _ _ _ _ _ _ _]
                    tunnel: [w450 w465 w472 w479 w495 w507 w525 w542 w619 w640 w674 w675 w690 w694 w707 w711] -> w374
                    tunnel: w355 -> [_ _ _ _ _ _ _ w540 w623 w637 _ _ _ _ _ _]
                    tunnel: w324 -> [w446 w467 w474 w481 w503 w510 w526 w545 w621 w644 w667 w687 w692 w696 w710 w712]
                    tunnel: w383 -> [_ _ _ _ _ w512 _ _ _ _ _ _ _ _ _ _]
                    tunnel: w395 -> [w448 w468 w475 w482 w494 w513 w522 w546 w617 w642 w672 w686 w693 w699 w709 w713]
                    tunnel: [w448 w468 w475 w482 w496 w511 w524 w546 w616 w641 w663 w679 w693 w697 w709 w713] -> w394
                    tunnel: w382 -> [_ _ _ _ _ _ _ w548 _ _ _ _ _ _ _ _]
                    tunnel: w381 -> [_ _ _ _ _ _ _ w547 _ _ _ _ _ _ _ _]
                    tunnel: [w450 w465 w472 w479 w495 w506 w525 w542 w619 w646 w674 w675 w690 w694 w707 w711] -> w373
                    tunnel: [w450 w465 w472 w479 w495 w506 w525 w542 w619 w645 w674 w675 w690 w694 w707 w711] -> w371
                    tunnel: [w447 w467 w474 w481 w503 w510 w526 w545 w620 w644 w667 w687 w692 w696 w710 w712] -> w386
                    tunnel: w302 -> [_ _ _ _ w486 _ _ w544 _ _ _ _ _ _ _ _]
                    tunnel: w392 -> [_ _ _ _ _ _ _ w543 _ _ _ _ _ _ _ _]
                    tunnel: w308 -> [_ _ _ _ _ _ _ _ _ w643 _ _ _ _ _ _]
                    tunnel: w391 -> [_ _ _ _ _ _ _ _ _ _ _ _ _ w698 _ _]
                    tunnel: [w450 w465 w472 w479 w495 w506 w525 w542 w619 w640 w674 TRUE w690 w694 w707 w711] -> w305
                    tunnel: w387 -> [_ _ _ _ _ _ _ _ _ _ _ w676 _ _ _ _]
                    tunnel: w345 -> [_ _ _ _ w500 _ _ _ _ _ _ _ _ _ _ _]
                    tunnel: w343 -> [_ _ _ _ _ _ _ _ _ _ w664 _ _ _ _ _]
                    tunnel: w306 -> [_ _ _ _ _ _ _ w537 _ w632 _ _ _ _ _ w715]
                    frame "idle", Default {
                      w450 = FALSE
                      n238 = local read "trialStart"() -> (w451:bool)
                      n239 = case shown="True" w451 {
                        tunnel: [w454 w457] -> w452
                        tunnel: w449 -> [w454 _]
                        tunnel: w446 -> [w453 w456]
                        tunnel: [w453 w455] -> w447
                        frame False {
                        }
                        frame True {
                          n240 = stacked-sequence {
                            tunnel: [w458 _] -> w457
                            tunnel: w456 -> [_ w464]
                            tunnel: [_ w463] -> w455
                            frame #0 {
                              n241 = local read "toneReward"() -> (w459:bool)
                              n242 = case shown="False" w459 {
                                tunnel: [states_def."tone" states_def."vs before"] -> w458
                                frame True {
                                }
                                frame False {
                                }
                              }
                            }
                            frame #1 {
                              w462 = FALSE
                              n243 = local write "trialStart"(w462) -> ()
                              n244 = local write "skipRewFlag"(w462) -> ()
                              n245 = Increment(x=w464) -> (x+1=w463:i32)
                            }
                          }
                        }
                      }
                    }
                    frame "vs before" {
                      w465 = FALSE
                      n246 = Select(t=states_def."vs", s=w471, f=w469) -> (s? t:f=w470:T5)
                    }
                    frame "vs" {
                      w472 = FALSE
                      n247 = Select(t=w477, s=w478, f=states_def."delay") -> (s? t:f=w476:T5)
                    }
                    frame "vs after" {
                      w479 = FALSE
                      n248 = Select(t=w485, s=w484, f=states_def."delay") -> (s? t:f=w483:T5)
                    }
                    frame "delay" {
                      w495 = FALSE
                      n249 = local read "allowPunish"() -> (w487:bool)
                      n250 = Not Equal?(x=w499, y=w498) -> (x != y?=w497:bool)
                      n251 = Select(t=w501, s=w497, f=w494) -> (s? t:f=w496:u64)
                      n252 = And(x=w487, y=w486) -> (x .and. y?=w488:bool)
                      n253 = case shown="True" w488 {
                        selector: w488 -> [_ w505]
                        frame False {
                        }
                        frame True {
                          n254 = local write "skipRewFlag"(w505) -> ()
                        }
                      }
                      n255 = Add(x=w500, y=w496) -> (x+y=w502:u64)
                      n256 = local read "skipRewFlag"() -> (w492:bool)
                      n257 = Less?(x=w502, y=w501) -> (x < y?=w493:bool)
                      n258 = Select(t=states_def."timeout", s=w492, f=states_def."tone after") -> (s? t:f=w490:T5)
                      n259 = Select(t=w490, s=w493, f=w498) -> (s? t:f=w504:T5)
                    }
                    frame "tone before" {
                      w506 = FALSE
                      n260 = case shown="True" w512 {
                        tunnel: [w517 states_def."tone after"] -> w508
                        tunnel: w514 -> [w517 _]
                        tunnel: w513 -> [w516 _]
                        tunnel: [w516 w520] -> w511
                        tunnel: w509 -> [_ w520]
                        tunnel: [TRUE FALSE] -> w507
                        frame False {
                        }
                        frame True {
                        }
                      }
                    }
                    frame "tone" {
                      w525 = FALSE
                      n261 = local read "Busy"() -> (w521:bool)
                      n262 = case shown="True" w521 {
                        tunnel: [w530 states_def."tone after"] -> w528
                        tunnel: w527 -> [w530 _]
                        tunnel: w523 -> [_ w531]
                        tunnel: [w529 w531] -> w524
                        tunnel: w522 -> [w529 _]
                        frame False {
                        }
                        frame True {
                        }
                      }
                    }
                    frame "tone after" {
                      w542 = FALSE
                      n263 = local read "toneReward"() -> (w539:bool)
                      n264 = local read "allowAutoWater"() -> (w535:bool)
                      n265 = Or(x=w539, y=w540) -> (x .or. y?=w538:bool)
                      n266 = case shown="True" w544 {
                        tunnel: w548 -> [_ w576]
                        tunnel: w547 -> [_ w575]
                        tunnel: w538 -> [_ w574]
                        tunnel: w537 -> [_ w573]
                        tunnel: [w565 w571] -> w534
                        tunnel: w536 -> [w565 w569]
                        frame False {
                        }
                        frame True {
                          n267 = case shown="True" w574 {
                            tunnel: [w592 w606] -> w566
                            tunnel: w576 -> [w589 w605]
                            tunnel: w575 -> [w593 w604]
                            tunnel: w573 -> [_ w603]
                            frame True {
                              n268 = Not(x=w589) -> (.not. x?=w594:bool)
                              n269 = Not(x=w593) -> (.not. x?=w590:bool)
                              n270 = local read "rightcounter"() -> (w586:i32)
                              n271 = local read "leftcounter"() -> (w587:i32)
                              n272 = Select(t=3, s="forceLRswitch", f=inf) -> (s? t:f=w577:dbl)
                              n273 = Select(t=3, s="forceLRswitch", f=inf) -> (s? t:f=w583:dbl)
                              n274 = Less?(x=w586, y=w577) -> (x < y?=w585:bool)
                              n275 = Compound Arithmetic op=AND(w594, w593, w585) -> (w591:bool)
                              n276 = Less?(x=w587, y=w583) -> (x < y?=w588:bool)
                              n277 = Compound Arithmetic op=AND(w588, w589, w590) -> (w584:bool)
                              n278 = case shown="True" w584 {
                                frame False {
                                }
                                frame True {
                                n279 = local read "leftcounter"() -> (w600:i32)
                                n280 = local write "FlagWaterLeft"(TRUE) -> ()
                                n281 = Increment(x=w600) -> (x+1=w601:i32)
                                n282 = local write "leftcounter"(w601) -> ()
                                n283 = local write "rightcounter"(0) -> ()
                                }
                              }
                              n284 = case shown="True" w591 {
                                frame False {
                                }
                                frame True {
                                n285 = local read "rightcounter"() -> (w596:i32)
                                n286 = local write "FlagWaterLeft"(FALSE) -> ()
                                n287 = Increment(x=w596) -> (x+1=w595:i32)
                                n288 = local write "rightcounter"(w595) -> ()
                                n289 = local write "leftcounter"(0) -> ()
                                }
                              }
                              n290 = Exclusive Or(1:w591, 2:w584) -> (0:w592:bool)
                            }
                            frame False {
                              # "Consider add another state for automaticaly give water \nwhen animal did not get water for consecutively 10 trials?"
                              n291 = case shown="2" w603 {
                                tunnel: [w609 w611] -> w606
                                tunnel: w605 -> [w608 w614]
                                tunnel: w604 -> [w607 w612]
                                frame 1, Default {
                                # "left"
                                n292 = Not(x=w607) -> (.not. x?=w610:bool)
                                n293 = And(x=w608, y=w610) -> (x .and. y?=w609:bool)
                                }
                                frame 2 {
                                # "right"
                                n294 = Not(x=w614) -> (.not. x?=w613:bool)
                                n295 = And(x=w613, y=w612) -> (x .and. y?=w611:bool)
                                }
                              }
                            }
                          }
                          n296 = local read "allowCorrection"() -> (w568:bool)
                          n297 = Select(t=w569, s=w568, f=states_def."timeout") -> (s? t:f=w567:T5)
                          n298 = Select(t=states_def."reward", s=w566, f=w567) -> (s? t:f=w571:T5)
                        }
                      }
                      n299 = case shown="True" w535 {
                        tunnel: w534 -> [w553 w563]
                        tunnel: [w553 w562] -> w533
                        frame False {
                        }
                        frame True {
                          w556 = 10 ("Priority")
                          n300 = local read "contNoReward"() -> (w560:i32)
                          n301 = Random Number (0-1)() -> (number: 0 to 1=w557:dbl)
                          n302 = Multiply(x=w557, y=w556) -> (x*y=w555:dbl)
                          n303 = Add(x=w555, y=w556) -> (x+y=w554:dbl)
                          n304 = Greater Or Equal?(x=w560, y=w554) -> (x >= y?=w559:bool)
                          n305 = Select(t=0 ("Priority"), s=w559, f=w560) -> (s? t:f=w558:i32)
                          n306 = Select(t=states_def."manualwater", s=w559, f=w563) -> (s? t:f=w562:T5)
                          n307 = local write "contNoReward"(w558) -> ()
                        }
                      }
                      n308 = Add(x=w543, y=w546) -> (x+y=w552:u64)
                      n309 = Greater?(x=w551, y=w552) -> (0:w549:bool)
                      n310 = Select(t=states_def."cycle end", s=w549, f=w533) -> (s? t:f=w550:T5)
                    }
                    frame "cycle end" {
                      w619 = FALSE
                      # "inform host computer to start \nanother trial"
                      n311 = case shown="False" w623 {
                        tunnel: [w624 w630] -> w620
                        tunnel: [states_def."idle" states_def."tone after"] -> w622
                        tunnel: w621 -> [w624 w630]
                        tunnel: [w625 w628] -> w616
                        tunnel: w618 -> [w625 w628]
                        tunnel: w617 -> [_ _]
                        tunnel: w615 -> [_ _]
                        frame False {
                          n312 = local write "trialDone"(TRUE) -> ()
                        }
                        frame True {
                        }
                      }
                    }
                    frame "reward" {
                      w640 = FALSE
                      n313 = Not Equal?(x=w652, y=w634) -> (x != y?=w647:bool)
                      n314 = local read "toneReward"() -> (w638:bool)
                      n315 = Select(t=w650, s=w647, f=w642) -> (s? t:f=w641:u64)
                      n316 = Or(x=w637, y=w638) -> (x .or. y?=w639:bool)
                      n317 = case shown="False" w639 {
                        tunnel: [w654 w657] -> w646
                        tunnel: [w653 w656] -> w645
                        tunnel: w632 -> [_ w655]
                        frame True {
                          n318 = local read "FlagWaterLeft"() -> (w654:bool)
                          n319 = Not(x=w654) -> (.not. x?=w653:bool)
                        }
                        frame False {
                          n320 = case shown="0, Default" w655 {
                            tunnel: [w658 w660 w661] -> w657
                            tunnel: [w658 w659 w662] -> w656
                            frame 0, Default {
                              w658 = FALSE
                            }
                            frame 1 {
                              w660 = TRUE
                              n321 = Not(x=w660) -> (.not. x?=w659:bool)
                            }
                            frame 2 {
                              w662 = TRUE
                              n322 = Not(x=w662) -> (.not. x?=w661:bool)
                            }
                          }
                        }
                      }
                      n323 = Add(x=w643, y=w641) -> (x+y=w651:u64)
                      n324 = Less?(x=w651, y=w650) -> (x < y?=w649:bool)
                      n325 = Select(t=states_def."reward refractory", s=w637, f=states_def."cycle end") -> (s? t:f=w633:T5)
                      n326 = local write "rewardStatus"(TRUE) -> ()
                      n327 = Select(t=w633, s=w649, f=w634) -> (s? t:f=w648:T5)
                    }
                    frame "reward refractory" {
                      w674 = FALSE
                      n328 = Not Equal?(x=w669, y=w669) -> (x != y?=w673:bool)
                      n329 = Select(t=w666, s=w673, f=w672) -> (s? t:f=w663:u64)
                      n330 = Add(x=w663, y=w664) -> (x+y=w665:u64)
                      n331 = Greater?(x=w666, y=w665) -> (0:w671:bool)
                      n332 = Select(t=states_def."cycle end", s=w671, f=w669) -> (s? t:f=w670:T5)
                    }
                    frame "punish" {
                      w675 = FALSE
                      n333 = Not Equal?(x=w683, y=w677) -> (x != y?=w685:bool)
                      n334 = case shown="True" w685 {
                        tunnel: w677 -> [_ w689]
                        frame False {
                        }
                        frame True {
                          "curState" <- w689
                        }
                      }
                      n335 = Select(t=w678, s=w685, f=w686) -> (s? t:f=w679:u64)
                      n336 = Add(x=w679, y=w676) -> (x+y=w680:u64)
                      n337 = Less?(x=w678, y=w680) -> (x < y?=w684:bool)
                      n338 = local read "curState"() -> (w682:u32)
                      n339 = Select(t=w677, s=w684, f=w682) -> (s? t:f=w681:u32)
                    }
                    frame "punish refractory" {
                      w690 = FALSE
                      # "To do"
                    }
                    frame "timeout" {
                      w694 = FALSE
                      # "To do: change the state when timeout finished?????"
                      n340 = Not Equal?(x=w703, y=w702) -> (x != y?=w706:bool)
                      n341 = Select(t=w700, s=w706, f=w699) -> (s? t:f=w697:u64)
                      n342 = Add(x=w697, y=w698) -> (x+y=w705:u64)
                      n343 = Greater?(x=w700, y=w705) -> (0:w704:bool)
                      n344 = Select(t=states_def."cycle end", s=w704, f=w702) -> (s? t:f=w701:T5)
                    }
                    frame "exit" {
                      w707 = FALSE
                    }
                    frame "manualwater" {
                      w711 = FALSE
                      n345 = case shown="1" w715 {
                        frame 0, Default {
                        }
                        frame 1 {
                          n346 = local write "manualWaterLeft"(TRUE) -> ()
                        }
                        frame 2 {
                          n347 = local write "manualWaterRight"(TRUE) -> ()
                        }
                      }
                    }
                  }
                  n348 = local read "rtFIFOdataPool"() -> (w351:u32)
                  n349 = local read "rtFIFOdataDim"() -> (w356:i32)
                  n350 = Multiply(x=w356, y=w351) -> (x*y=w357:u32)
                  n351 = local read "manualWaterRight"() -> (w312:bool)
                  n352 = case shown="False" w312 {
                    tunnel: [w409 w418] -> w310
                    tunnel: w311 -> [w410 _]
                    tunnel: w309 -> [w408 w418]
                    tunnel: w308 -> [w407 _]
                    frame False {
                      n353 = local read "rightWaterOnFlag"() -> (w406:bool)
                      n354 = case shown="True" w406 {
                        tunnel: w410 -> [_ w415]
                        tunnel: [0 w415] -> w409
                        tunnel: w408 -> [_ w417]
                        tunnel: w407 -> [_ w416]
                        frame False {
                        }
                        frame True {
                          n355 = Add(x=w416, y=w415) -> (x+y=w414:u64)
                          n356 = Greater?(x=w417, y=w414) -> (0:w413:bool)
                          n357 = Not(x=w413) -> (.not. x?=w412:bool)
                          n358 = local write "rightWaterOnFlag"(w412) -> ()
                        }
                      }
                    }
                    frame True {
                      n359 = local write "manualWaterRight"(FALSE) -> ()
                      n360 = local write "rightWaterOnFlag"(TRUE) -> ()
                    }
                  }
                  n361 = shared-variable ".\\variables - network - RT (separate).lvlib\\stop - network"() -> (w403:bool)  [unwired: 1 in, 1 out]
                  n362 = local read "leftWaterOnFlag"() -> (w313:bool)
                  n363 = local read "rightWaterOnFlag"() -> (w307:bool)
                  n364 = local read "manualShock"() -> (w304:bool)
                  n365 = local read "allowPunish"() -> (w303:bool)
                  n366 = Select(t=states_def."exit", s=w403, f=w301) -> (s? t:f=w393:u32)
                  n367 = feedback-in #2(w393) -> ()
                  n368 = feedback-in #3(w393) -> ()
                  n369 = call "punish_check.vi"("input state"=w301, "lick"=w302, "allow punish"=w303) -> ("punish"=w300:bool)
                  n370 = Or(x=w313, y=w373) -> (x .or. y?=w372:bool)
                  n371 = Or(x=w307, y=w371) -> (x .or. y?=w370:bool)
                  n372 = Compound Arithmetic op=OR(w300, w304, w305) -> (w390:bool)
                  n373 = local read "ABORT"() -> (w337:bool)
                  n374 = Build Array(w374, w372, w370, w390) -> (w366:bool[])
                  n375 = Build Array (concatenate)(w369, w366, w368) -> (w367:bool[])
                  n376 = Boolean Array To Number(Boolean array=w367) -> (number=w319:u32)
                  n377 = Build Array (concatenate)(w360, w319, w317) -> (w358:dbl[])
                  n378 = Array Size(array=w358) -> (size(s)=w339:i32)
                  n379 = Build Array (concatenate)(w380, w358) -> (w378:dbl[])
                  n380 = local write "rtFIFOdataDim"(w339) -> ()
                  n381 = Array Size(array=w378) -> (size(s)=w375:i32)
                  n382 = Equal?(x=w375, y=w357) -> (x = y?=w377:bool)
                  n383 = Not Equal?(x=w339, y=9) -> (x != y?=w338:bool)
                  n384 = case shown="True" w377 {
                    tunnel: [w438 w445] -> w376
                    tunnel: w378 -> [w439 w442]
                    tunnel: [w439 sgl[] [] ("array type (2D Dbl)")] -> w379
                    tunnel: w353 -> [_ w441]
                    tunnel: w352 -> [w438 w440]
                    frame False {
                    }
                    frame True {
                      n385 = local read "rtFIFOtimeout"() -> (w443:u32)
                      n386 = RT FIFO Write(0:w441, 1:w442, 2:w443, 3:w440) -> (11:w445:errorcluster)  [unwired: 1 in, 3 out]
                    }
                  }
                  n387 = case shown="True" w338 {
                    frame False {
                    }
                    frame True {
                      n388 = One Button Dialog(message="The dimention of rtFIFOdata is not 4, pleae change the size of alocated network stream.") -> (true=w436:bool)  [unwired: 1 in]
                      n389 = local write "ABORT"(w436) -> ()
                    }
                  }
                  n390 = call-poly <vilib>:"DAQmx Write.vi"("task/channels in"=w342, "data"=w366, "error in"=w341) -> ("task out"=w397:refnum<k21>, "error out"=w396:errorcluster)  [unwired: 10 in, 1 out]
                  n391 = node-c288() -> ()  [unwired: 1 in, 1 out]
                }
                n392 = node-c288(5.0, 100 ("Priority")) -> (w230:T2)  [unwired: 1 in]
                n393 = timed-loop {
                  timing: w230 -> [_]
                  timing-out: [_] -> w229
                  tunnel: [w270] -> w207
                  tunnel: [w269] -> w206
                  tunnel: [w268] -> w209
                  tunnel: [w267] -> w208
                  tunnel: w228 -> [w266]
                  tunnel: w227 -> [w265]
                  tunnel: w214 -> [w264]
                  tunnel: w213 -> [w263]
                  shift-right: [w273] -> _
                  shift-left: w223 -> [w272]
                  stop <- w271 stop-if-true
                  n394 = node-c288() -> ()  [unwired: 1 in, 1 out]
                  n395 = property class="Network Stream Endpoint"(reference=w265, error in=w266) -> (reference out=w275:refnum<k21>, error out=w274:errorcluster, "Connected"=→"Is Connected":bool, "AvailElmntsForWrite"=→"Available Elements for Writing":i32)
                  n396 = RT FIFO Read(0:w264, 2:0, 3:w263) -> (8:w268:refnum<k33>, 9:w261:sgl[], 11:w267:errorcluster)  [unwired: 1 in, 2 out]
                  n397 = Empty Array?(array=w261) -> (empty?=w260:bool)
                  n398 = case shown="True" w260 {
                    tunnel: w261 -> [w283 _]
                    tunnel: [FALSE w288] -> w271
                    tunnel: w275 -> [w285 w286]
                    tunnel: w274 -> [w284 w287]
                    tunnel: [w278 w289] -> w273
                    tunnel: w272 -> [w281 w289]
                    tunnel: [w280 w286] -> w270
                    tunnel: [w279 w287] -> w269
                    frame False {
                      n399 = Increment(x=w281) -> (x+1=w278:i32)
                      n400 = shared-variable-write(w285, w284, w283) -> (w280:refnum<k21>, w279:errorcluster)  [unwired: 1 in, 1 out]
                      n401 = local write "stream counter"(w278) -> ()
                    }
                    frame True {
                      n402 = local read "ABORT"() -> (w288:bool)
                    }
                  }
                  n403 = node-c288() -> ()  [unwired: 1 in, 1 out]
                }
                n404 = node-c288(w229) -> (w197:errorcluster)
                n405 = node-c288(w233) -> (w199:errorcluster)
                n406 = Flush Stream(8:w206, 11:w207) -> (0:w205:errorcluster, 3:w204:refnum<k21>)  [unwired: 2 in, 1 out]
                n407 = RT FIFO Delete(0:w209, 3:w208) -> (11:w202:errorcluster)  [unwired: 1 in]
                n408 = Destroy Stream Endpoint(8:w205, 11:w204) -> (0:w203:errorcluster)
                n409 = node-c288(w231) -> (w198:errorcluster)
                n410 = stacked-sequence {
                  tunnel: w203 -> [w241]
                  tunnel: [w241] -> w196
                  frame #0 {
                    n411 = shared-variable "Sabrina-RT1\\variables - network - RT (separate).lvlib\\stop - network"(TRUE ("stop - network")) -> ()  [unwired: 1 in, 1 out]
                  }
                }
                n412 = Build Array(w194, w194, w194, w194) -> (w193:bool[])
                n413 = call-poly <vilib>:"DAQmx Write.vi"("task/channels in"=w201, "data"=w193, "error in"=w200) -> ("task out"=w174:refnum<k21>, "error out"=w173:errorcluster)  [unwired: 10 in, 1 out]
                n414 = call <vilib>:"DAQmx Stop Task.vi"("task/channels in"=w176, "error in"=w175) -> ("error out"=w172:errorcluster)  [unwired: 12 in, 1 out]
                n415 = call <vilib>:"DAQmx Stop Task.vi"("task/channels in"=w174, "error in"=w173) -> ("error out"=w171:errorcluster)  [unwired: 12 in, 1 out]
                n416 = Merge Errors(w191, w202) -> (w195:errorcluster)
                n417 = Merge Errors(w172, w171) -> (w177:errorcluster)
                n418 = Merge Errors(w199, w198, w197) -> (w178:errorcluster)
                n419 = Merge Errors(w178, w177, w195, w196) -> (w192:errorcluster)
                "error out" <- w192
                n420 = call <vilib>:"Simple Error Handler.vi"("error in (no error)"=w192) -> ()  [unwired: 4 in, 5 out]
              }
            }
          }
          frame #2 {
            n421 = Wait (ms)(milliseconds to wait=u32 100) -> ()  [unwired: 1 out]
          }
        }
      }
      n422 = UDP Close(connection ID=w23, 8:w22) -> (error out=w24:errorcluster)  [unwired: 1 out]
      n423 = UDP Close(connection ID=w18, 8:w19) -> (error out=w17:errorcluster)  [unwired: 1 out]
      n424 = call <vilib>:"Simple Error Handler.vi"("error in (no error)"=w24) -> ()  [unwired: 4 in, 5 out]
      n425 = call <vilib>:"Simple Error Handler.vi"("error in (no error)"=w17) -> ()  [unwired: 4 in, 5 out]
    }
  }
